vi "FancySliderUpdateByRef.vi"(8 "Error In":errorcluster, 10 "IMU in":T1 {"Gyroscope"."Z" scale=-45.0..45.0; "Gyroscope"."Y" scale=-45.0..45.0; "Gyroscope"."X" scale=-45.0..45.0; "Magnetometer"."Z" scale=-2500.0..2500.0; "Magnetometer"."Y" scale=-2500.0..2500.0; "Magnetometer"."X" scale=-2500.0..2500.0; "Accelerometer"."Z" scale=-5.0..5.0; "Accelerometer"."Y" scale=-5.0..5.0; "Accelerometer"."X" scale=-5.0..5.0}, 11 "IMU Ref":refnum<vi>) -> (0 "Error Out":errorcluster, 3 "IMU":T1 {"Gyroscope"."Z" scale=-45.0..45.0; "Gyroscope"."Y" scale=-45.0..45.0; "Gyroscope"."X" scale=-45.0..45.0; "Magnetometer"."Z" scale=-2500.0..2500.0; "Magnetometer"."Y" scale=-2500.0..2500.0; "Magnetometer"."X" scale=-2500.0..2500.0; "Accelerometer"."Z" scale=-5.0..5.0; "Accelerometer"."Y" scale=-5.0..5.0; "Accelerometer"."X" scale=-5.0..5.0})   [LabVIEW 2017]
uses:
  IMU Control.ctl
panel:
  out "Label.Text 2":string
  out "Label.Text":string
  out "Array":string[][](array[string])
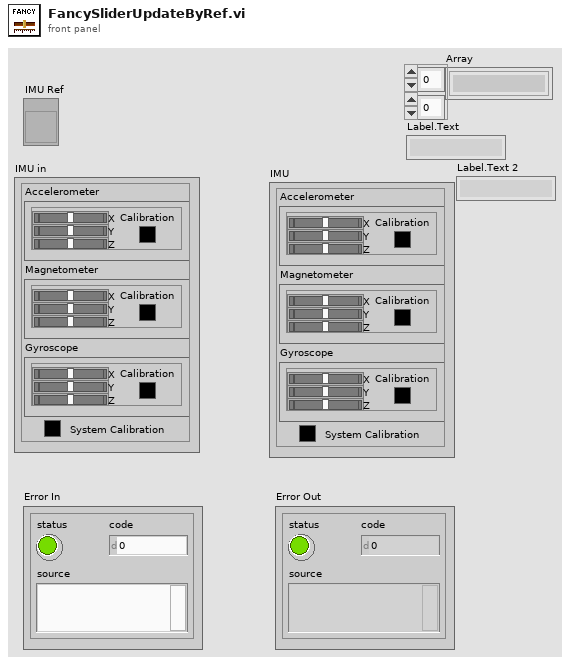
[diagram p1: front panel]
types:
  T1 = typedef "IMU Control.ctl" = cluster{"Accelerometer":cluster{"X":dbl, "Y":dbl, "Z":dbl, "Calibration":u32}, "Magnetometer":cluster{"X":dbl, "Y":dbl, "Z":dbl, "Calibration":u32}, "Gyroscope":cluster{"X":dbl, "Y":dbl, "Z":dbl, "Calibration":u32}, "System Calibration":u32}
  T2 = cluster{"X":dbl, "Y":dbl, "Z":dbl, "Calibration":u32}
  T3 = cluster{"X":dbl, "Y":dbl, "Z":dbl, "Calibration":u32}[]
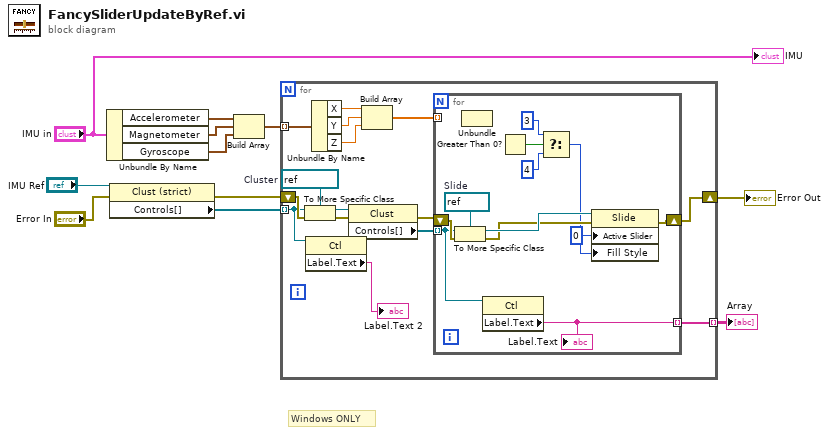
[diagram p0: block diagram]
diagram:
  # "Windows ONLY"
  n1 = Unbundle By Name("IMU in") -> ("Accelerometer"=w11:T2, "Magnetometer"=w10:T2, "Gyroscope"=w9:T2)
  n2 = property class="Clust (strict)"(reference="IMU Ref", error in="Error In") -> (error out=w6:errorcluster, "Controls[]"=w7:refnum<vi>[])  [unwired: 1 out]
  n3 = Build Array(w11, w10, w9) -> (w8:T3)
  n4 = for {
    tunnel: w8 -> [w24] mode=indexing
    tunnel: w7 -> [w13] mode=indexing
    shift-right: [w15] -> w4
    shift-left: w6 -> [w23]
    tunnel: [w14] -> w2 mode=indexing
    w25 = refnum<vi> refnum  # Cluster
    n5 = To More Specific Class(target class=w25, reference=w13, error in=w23) -> (specific class reference=w22:refnum<vi>, error out=w26:errorcluster)
    n6 = property class="Ctl"(reference=w13) -> ("Label.Text"=→"Label.Text 2":string)  [unwired: 1 in, 2 out]
    n7 = Unbundle By Name(w24) -> ("X"=w20:dbl, "Y"=w18:dbl, "Z"=w19:dbl)
    n8 = property class="Clust"(reference=w22, error in=w26) -> (error out=w16:errorcluster, "Controls[]"=w21:refnum<vi>[])  [unwired: 1 out]
    n9 = Build Array(w20, w18, w19) -> (w17:dbl[])
    n10 = for {
      tunnel: w21 -> [w30] mode=indexing
      tunnel: w17 -> [_] mode=indexing
      shift-right: [w31] -> w15
      shift-left: w16 -> [w38]
      tunnel: [w29] -> w14 mode=indexing
      w37 = refnum<vi> refnum  # Slide
      n11 = To More Specific Class(target class=w37, reference=w30, error in=w38) -> (specific class reference=w36:refnum<vi>, error out=w35:errorcluster)
      n12 = Unbundle() -> ()  [unwired: 1 in, 2 out]
      n13 = property class="Ctl"(reference=w30) -> ("Label.Text"=w29:string)  [unwired: 1 in, 2 out]
      "Label.Text" <- w29
      n14 = Greater Than 0?() -> (x > 0?=w28:bool)  [unwired: 1 in]
      n15 = Select(t=3 ("Fill Style"), s=w28, f=4 ("Fill Style")) -> (s? t:f=w32:i32)
      n16 = property class="Slide"(reference=w36, error in=w35, "Active Slider"=0, "Fill Style"=w32) -> (error out=w31:errorcluster)  [unwired: 1 out]
    }
  }
  "Error Out" <- w4
  "Array" <- w2
  "IMU" <- "IMU in"
